vi "4 DDS 8SPC.vi"(7 "clear DDS":bool, 8 "input valid":bool=TRUE, 9 "pdw in":T2 {"frequency shift" format="%#_12f"}, 10 "free DDS before me?":bool, 11 "new PDW in":bool) -> (0 "output valid":bool, 1 "state of every DDS":bool[](array[boolean]), 2 "have free DDS":bool, 3 "IQ out":T1[](array[typedef]))   [LabVIEW 2021]
doc: "transmit pulse with one free DDS inside.\nmust have no DDS before him (the distribute is to give the lowest mun DDS the pulse)"
uses:
  pulse_tx_vis/pdw.ctl
  pulse_tx_vis/CTL/mode_type.ctl
  <instrlib>/_niInstr/DSP/v1/Shared/Public/IQ Data.ctl
  <instrlib>/_niInstr/DSP/v1/Shared/niInstr DSP v1 Shared.lvlib
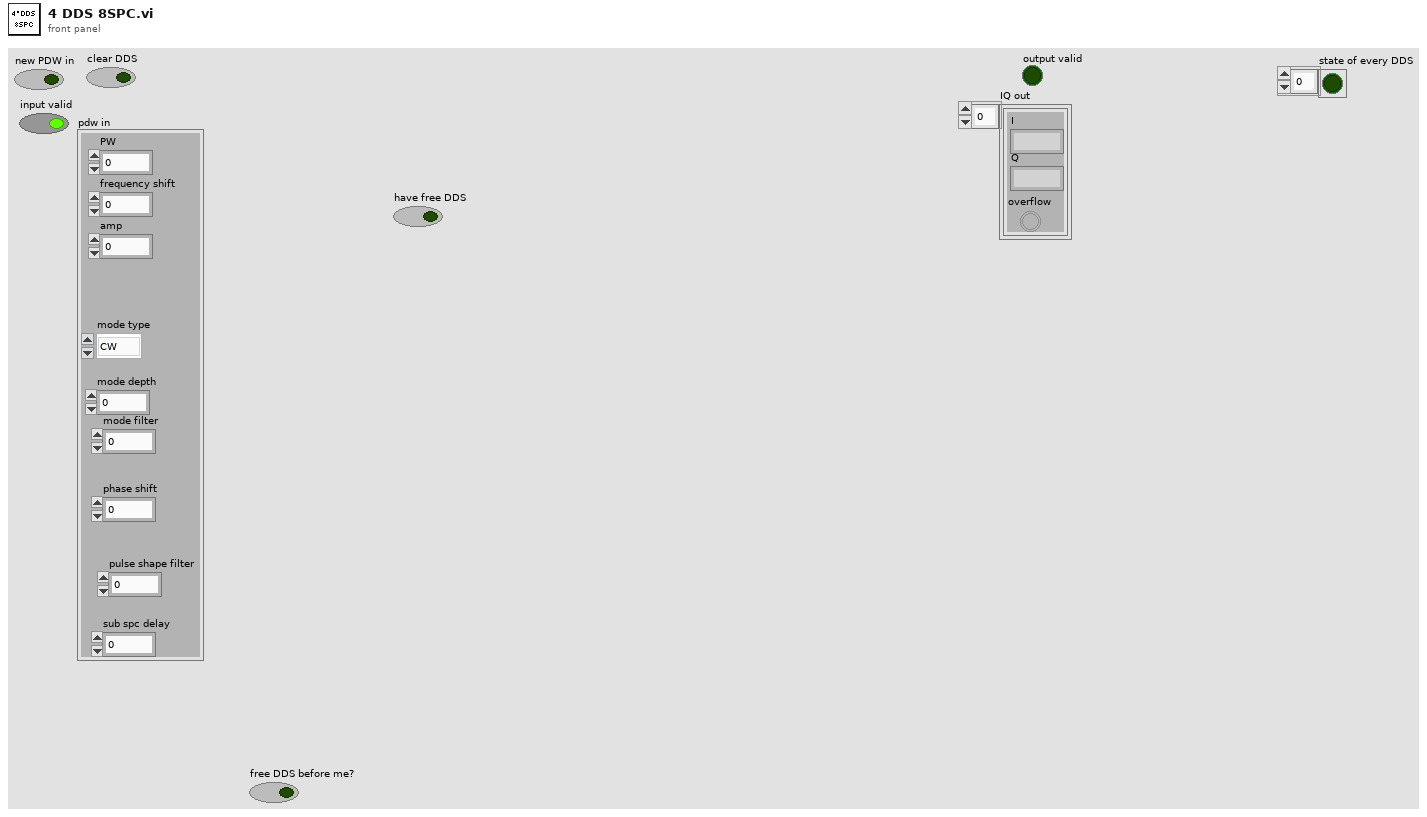
[diagram p1: front panel]
types:
  T1 = typedef "niInstr DSP v1 Shared.lvlib/IQ Data.ctl" = cluster{"I":fxp<+/-,18,1>, "Q":fxp<+/-,18,1>, "overflow":bool}
  T2 = typedef "pdw.ctl" = cluster{"PW":u32, "frequency shift":fxp<+/-,48,0>, "amp":fxp<+/-,18,1>, "mode type":T3, "mode depth":u32, "mode filter":u8, "phase shift":fxp<+/-,16,1>, "pulse shape filter":u8, "sub spc delay":u8}
  T3 = typedef "mode_type.ctl" = enum8{"CW", "from memory 1", "NC - cw", "LFM", "BPSK", "QPSK"}
  T4 = cluster{"I":fxp<+/-,18,1>, "Q":fxp<+/-,18,1>, "overflow":bool}[]
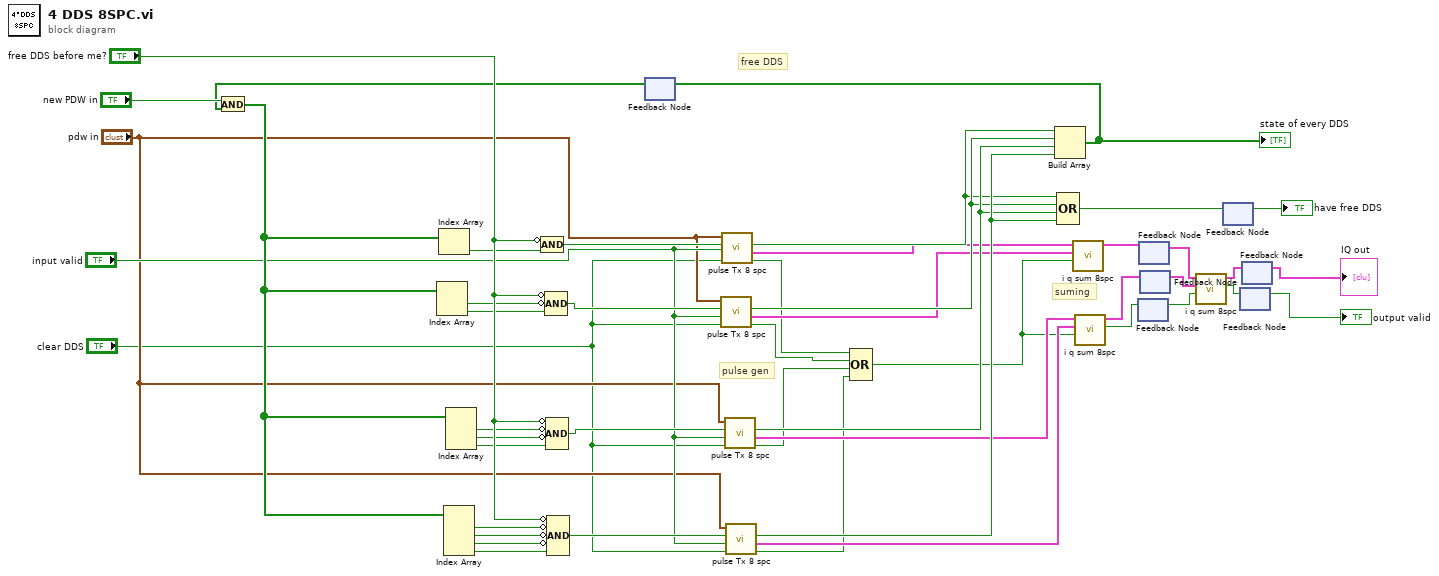
[diagram p0: block diagram]
diagram:
  # "free DDS"
  # "suming"
  # "pulse gen"
  n1 = feedback #1() -> (w22:bool[])  [unwired: 1 in]
  n2 = And(x="new PDW in", y=w22) -> (x .and. y?=w21:bool[])
  n3 = Index Array(array=w21) -> (element #1=w33:bool, element #2=w31:bool)  [unwired: 2 in]
  n4 = Index Array(array=w21) -> (element=w29:bool)  [unwired: 1 in]
  n5 = Index Array(array=w21) -> (element #1=w41:bool, element #2=w40:bool, element #3=w39:bool, element #4=w38:bool)  [unwired: 4 in]
  n6 = Index Array(array=w21) -> (element #1=w37:bool, element #2=w36:bool, element #3=w35:bool)  [unwired: 3 in]
  n7 = Compound Arithmetic op=AND(invert "free DDS before me?", w29) -> (w30:bool)
  n8 = Compound Arithmetic op=AND(invert "free DDS before me?", invert w33, w31) -> (w32:bool)
  n9 = Compound Arithmetic op=AND(invert "free DDS before me?", invert w37, invert w36, w35) -> (w34:bool)
  n10 = Compound Arithmetic op=AND(invert "free DDS before me?", invert w41, invert w40, invert w39, w38) -> (w42:bool)
  n11 = call "pulse Tx 8 spc.vi"("clear DDS"="clear DDS", "enable line"="input valid", "take it!"=w32, "Cluster"="pdw in") -> ("output valid"=w15:bool, "IQ out"=w26:T1[], "free dds"=w44:bool)  [unwired: 3 in, 2 out]
  n12 = call "pulse Tx 8 spc.vi"("clear DDS"="clear DDS", "enable line"="input valid", "take it!"=w30, "Cluster"="pdw in") -> ("output valid"=w16:bool, "IQ out"=w25:T1[], "free dds"=w43:bool)  [unwired: 3 in, 2 out]
  n13 = call "pulse Tx 8 spc.vi"("clear DDS"="clear DDS", "enable line"="input valid", "take it!"=w34, "Cluster"="pdw in") -> ("output valid"=w14:bool, "IQ out"=w27:T1[], "free dds"=w45:bool)  [unwired: 3 in, 2 out]
  n14 = call "pulse Tx 8 spc.vi"("clear DDS"="clear DDS", "enable line"="input valid", "take it!"=w42, "Cluster"="pdw in") -> ("output valid"=w13:bool, "IQ out"=w28:T1[], "free dds"=w46:bool)  [unwired: 3 in, 2 out]
  n15 = Compound Arithmetic op=OR(w16, w15, w14, w13) -> (w12:bool)
  n16 = Build Array(w43, w44, w45, w46) -> (w24:bool[])
  "state of every DDS" <- w24
  n17 = feedback-in #1(w24) -> ()
  n18 = Compound Arithmetic op=OR(w43, w44, w45, w46) -> (w20:bool)
  n19 = call "i q sum 8spc.vi"("input valid"=w12, "IQ in 2"=w26, "IQ in"=w25) -> ("IQ out"=w11:T4)  [unwired: 7 in, 1 out]
  n20 = call "i q sum 8spc.vi"("input valid"=w12, "IQ in 2"=w28, "IQ in"=w27) -> ("output valid"=w9:bool, "IQ out"=w10:T4)  [unwired: 7 in]
  n21 = feedback-in #2(w9) -> ()
  n22 = feedback #2() -> (w8:bool)  [unwired: 1 in]
  n23 = feedback #3() -> (w6:T4)  [unwired: 1 in]
  n24 = feedback-in #3(w11) -> ()
  n25 = feedback #4() -> (w7:T4)  [unwired: 1 in]
  n26 = feedback-in #4(w10) -> ()
  n27 = call "i q sum 8spc.vi"("input valid"=w8, "IQ in 2"=w7, "IQ in"=w6) -> ("output valid"=w3:bool, "IQ out"=w5:T4)  [unwired: 7 in]
  n28 = feedback #5() -> (→"have free DDS":bool)  [unwired: 1 in]
  n29 = feedback-in #5(w20) -> ()
  n30 = feedback #6() -> (→"output valid":bool)  [unwired: 1 in]
  n31 = feedback-in #6(w3) -> ()
  n32 = feedback #7() -> (→"IQ out":T4)  [unwired: 1 in]
  n33 = feedback-in #7(w5) -> ()
